vi "Bin-Digit.vi"(1 "b3":bool, 2 "b2":bool, 3 "b1":bool, 4 "b0":bool) -> (0 "Digit":i32)   [LabVIEW 2012]
panel:
  # "0"
  # "1"
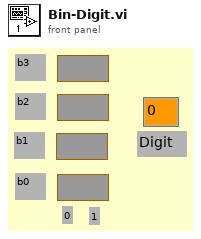
[diagram p1: front panel]
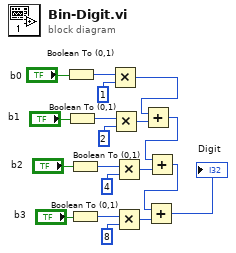
[diagram p0: block diagram]
diagram:
  n1 = Boolean To (0,1)(Boolean="b0") -> (0, 1=w18:i16)
  n2 = Boolean To (0,1)(Boolean="b1") -> (0, 1=w16:i16)
  n3 = Boolean To (0,1)(Boolean="b2") -> (0, 1=w14:i16)
  n4 = Boolean To (0,1)(Boolean="b3") -> (0, 1=w12:i16)
  n5 = Multiply(x=w18, y=1) -> (x*y=w5:i32)
  n6 = Multiply(x=w16, y=2) -> (x*y=w10:i32)
  n7 = Multiply(x=w14, y=4) -> (x*y=w8:i32)
  n8 = Multiply(x=w12, y=8) -> (x*y=w6:i32)
  n9 = Add(x=w5, y=w10) -> (x+y=w9:i32)
  n10 = Add(x=w9, y=w8) -> (x+y=w7:i32)
  n11 = Add(x=w7, y=w6) -> (x+y=→"Digit":i32)
